vi "TPISetPosition.vi"(0 "Current Position (µm)":cluster{"x":dbl, "y":dbl, "z":dbl} {"z" format="%.2f"; "y" format="%.2f"; "x" format="%.2f"}) -> ()   [LabVIEW 2009]
uses:
  <vilib>/Daq/1easyio.llb/AO Update Channels (scaled array).vi
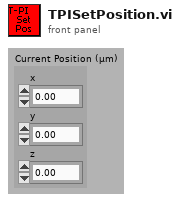
[diagram p1: front panel]
types:
  T1 = typedef "StageSettings.ctt" = cluster{"channels (x, y, z)":tag, "Stage Scaling (V/µm)":dbl}
  T2 = typedef "AnalogSettings.ctt" = cluster{"PCI 671x Device Number":u32, "Samples per Unit":u32}
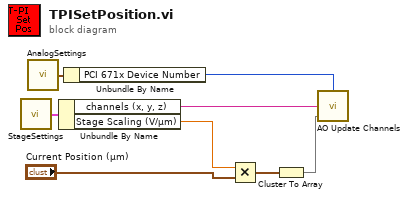
[diagram p0: block diagram]
diagram:
  n1 = call "StageSettings.vi"() -> ("PI Stage Setup (output)"=w7:T1)  [unwired: 2 in]
  n2 = call "AnalogSettings.vi"() -> ("Analog Settings (output)"=w5:T2)  [unwired: 2 in]
  n3 = Unbundle By Name(w7) -> ("channels (x, y, z)"=w8:tag, "Stage Scaling (V/µm)"=w3:dbl)
  n4 = Unbundle By Name(w5) -> ("PCI 671x Device Number"=w4:u32)
  n5 = Multiply(x=w3, y="Current Position (µm)") -> (x*y=w1:cluster{"x":dbl, "y":dbl, "z":dbl})
  n6 = Cluster To Array(cluster=w1) -> (array=w6:dbl[])
  n7 = call-poly <vilib>:"AO Update Channels.vi"("values"=w6, "channels (0)"=w8, "device"=w4) -> ()
